vi "LSI336Data_initialize.vi"(0 "LSI336Data in":refnum<class "LSI336Data.lvclass">, 1 "RunName":string, 2 "InstName":string, 3 "FileFormat":string, 5 "LSI336Settings(X, Y)":T2(array[cluster])=[{"LSIName"="LSI218A", "Labels"=["N.C.", "N.C.", "N.C.", "N.C.", "N.C.", "N.C.", "N.C.", "N.C."], "SensorLocations"=[enum."N.C.", enum."N.C.", enum."N.C.", enum."N.C.", enum."N.C.", enum."N.C.", enum."N.C.", enum."N.C."], "Active?"=FALSE, "VISA res. name"=""}, {"LSIName"="LSI218B", "Labels"=["N.C.", "N.C.", "N.C.", "N.C.", "N.C.", "N.C.", "N.C.", "N.C."], "SensorLocations"=[enum."N.C.", enum."N.C.", enum."N.C.", enum."N.C.", enum."N.C.", enum."N.C.", enum."N.C.", enum."N.C."], "Active?"=FALSE, "VISA res. name"=""}, {"LSIName"="LSI218C", "Labels"=["N.C.", "N.C.", "N.C.", "N.C.", "N.C.", "N.C.", "N.C.", "N.C."], "SensorLocations"=[enum."N.C.", enum."N.C.", enum."N.C.", enum."N.C.", enum."N.C.", enum."N.C.", enum."N.C.", enum."N.C."], "Active?"=FALSE, "VISA res. name"=""}, {"LSIName"="LSI218D", "Labels"=["N.C.", "N.C.", "N.C.", "N.C.", "N.C.", "N.C.", "N.C.", "N.C."], "SensorLocations"=[enum."N.C.", enum."N.C.", enum."N.C.", enum."N.C.", enum."N.C.", enum."N.C.", enum."N.C.", enum."N.C."], "Active?"=FALSE, "VISA res. name"=""}, {"LSIName"="LSI218E", "Labels"=["N.C.", "N.C.", "N.C.", "N.C.", "N.C.", "N.C.", "N.C.", "N.C."], "SensorLocations"=[enum."N.C.", enum."N.C.", enum."N.C.", enum."N.C.", enum."N.C.", enum."N.C.", enum."N.C.", enum."N.C."], "Active?"=FALSE, "VISA res. name"=""}, {"LSIName"="LSI218F", "Labels"=["N.C.", "N.C.", "N.C.", "N.C.", "N.C.", "N.C.", "N.C.", "N.C."], "SensorLocations"=[enum."N.C.", enum."N.C.", enum."N.C.", enum."N.C.", enum."N.C.", enum."N.C.", enum."N.C.", enum."N.C."], "Active?"=FALSE, "VISA res. name"=""}], 9 "RUN start time":timestamp, 11 "error in (no error)":errorcluster, 12 "base path":path) -> (4 "LSI336Data out":refnum<class "LSI336Data.lvclass">, 6 "Status":T1(ring), 10 "AllLabels":string[](array[string]), 15 "error out":errorcluster)   [LabVIEW 2017, in "LSI336Data.lvclass"]
uses:
  LSI336Data.lvclass
  LSI336Data.lvclass/LSI336Data.ctl
  istr.lib/Lake Shore 336/Lake Shore 336.lvlib
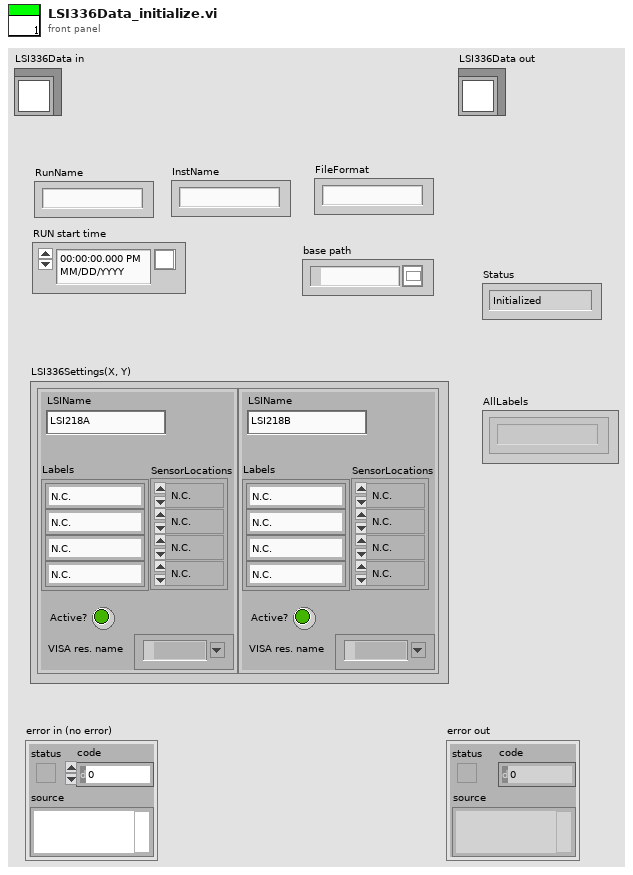
[diagram p1: front panel]
types:
  T1 = enum16{"Initialized", "Ready", "Measuring", "Terminated"}
  T2 = cluster{"LSIName":string, "Labels":string[], "SensorLocations":enum16{"N.C.", "T3He1-1", "T3He1-2", "T3He1-3", "T3He1-4", "T3He2-1", "T3He2-2", "T3He3", "T3He4", "T3He5", "T3He6-1", "T3He6-2", "T3He7-1", "T3He7-2", "T3He8", "T3He9", "T3He10", "T4He1", "T4He2-1", "T4He2-2", "T4He3-1", "T4He3-2", "T4He3-3", "T4He3-4", "T4He4", "T4He5", "T4He6", "T4He7", "T4He8", "T4He9", "T4He10", "T1K1", "T1K2", "T1K3-1", "T1K3-2", "T1K4", "T1K5", "T1K6", "TIP1", "TIP2", "TIP3", "TIP4", "TIP5", "TIP6", "TIP7", "TTH1", "TTH2", "TTH3", "TTH4"}[], "Active?":bool, "VISA res. name":refnum<visa-resource-name>}[]
  T3 = enum16{"open", "replace", "create", "open or create", "replace or create", "replace or create with confirmation"}
  T4 = cluster{"LSIName":string, "Labels":string[], "SensorLocations":enum16{"N.C.", "T3He1-1", "T3He1-2", "T3He1-3", "T3He1-4", "T3He2-1", "T3He2-2", "T3He3", "T3He4", "T3He5", "T3He6-1", "T3He6-2", "T3He7-1", "T3He7-2", "T3He8", "T3He9", "T3He10", "T4He1", "T4He2-1", "T4He2-2", "T4He3-1", "T4He3-2", "T4He3-3", "T4He3-4", "T4He4", "T4He5", "T4He6", "T4He7", "T4He8", "T4He9", "T4He10", "T1K1", "T1K2", "T1K3-1", "T1K3-2", "T1K4", "T1K5", "T1K6", "TIP1", "TIP2", "TIP3", "TIP4", "TIP5", "TIP6", "TIP7", "TTH1", "TTH2", "TTH3", "TTH4"}[], "Active?":bool, "VISA res. name":refnum<visa-resource-name>}
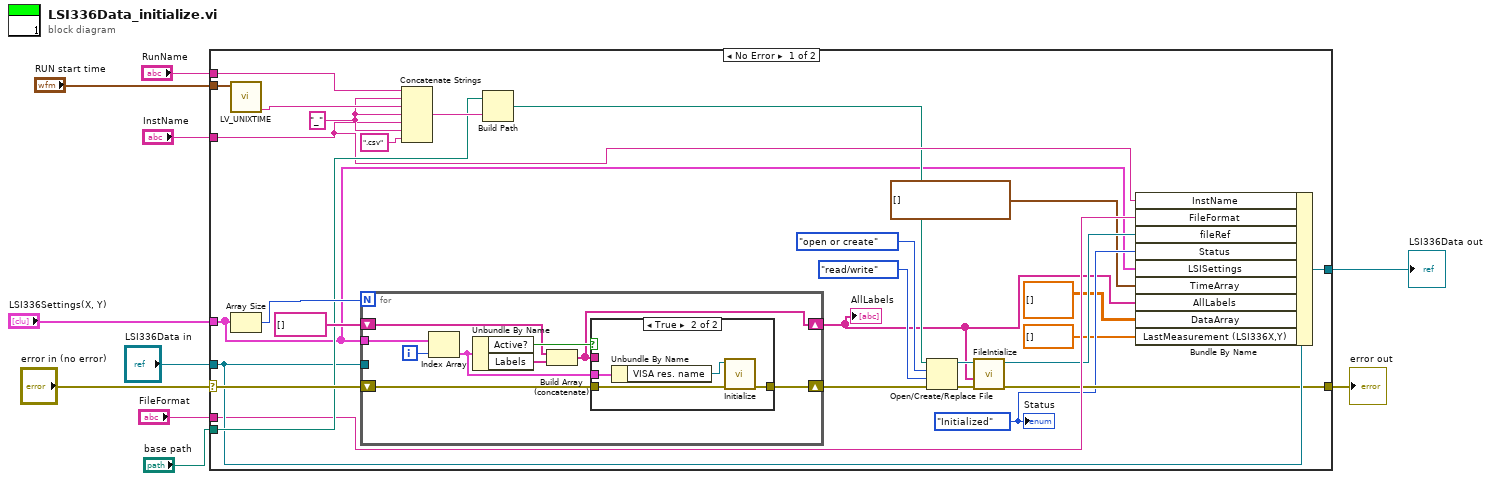
[diagram p0: block diagram]
diagram:
  n1 = case shown="No Error" "error in (no error)" {
    selector: "error in (no error)" -> [w38 w54]
    tunnel: [w20 w54] -> w9
    tunnel: [w17 w53] -> w7
    tunnel: "LSI336Data in" -> [w27 w53]
    tunnel: "LSI336Settings(X, Y)" -> [w15 _]
    tunnel: "RunName" -> [w34 _]
    tunnel: "RUN start time" -> [w33 _]
    tunnel: "InstName" -> [w26 _]
    tunnel: "base path" -> [w28 _]
    tunnel: "FileFormat" -> [w25 _]
    frame No Error {
      w16 = T1."Initialized" ("Status")
      w31 = "_" ("string")
      n2 = call "LV_UNIXTIME.vi"("current time"=w33) -> ("date/time string"=w32:string)  [unwired: 9 in, 1 out]
      n3 = Array Size(array=w15) -> (size(s)=w36:i32)
      n4 = for {
        N: w36 -> [_]
        shift-right: [w42] -> w14
        shift-left: string[] [] -> [w43]
        shift-right: [w39] -> w35
        shift-left: w38 -> [w40]
        tunnel: w27 -> [_]
        tunnel: w15 -> [w46]
        i -> [w47]
        n5 = Index Array(array=w46, index=w47) -> (element=w41:T4)
        n6 = Unbundle By Name(w41) -> ("Active?"=w45:bool, "Labels"=w44:string[])
        n7 = Build Array (concatenate)(w43, w44) -> (w42:string[])
        n8 = case shown="True" w45 {
          tunnel: w42 -> [_ _]
          tunnel: w41 -> [_ w51]
          tunnel: w40 -> [w48 w50]
          tunnel: [w48 w49] -> w39
          frame False {
          }
          frame True {
            n9 = Unbundle By Name(w51) -> ("VISA res. name"=w52:refnum<visa-resource-name>)
            n10 = call "Initialize.vi"("error in (no error)"=w50, "VISA resource name"=w52) -> ("error out"=w49:errorcluster)  [unwired: 8 in, 1 out]
          }
        }
      }
      "AllLabels" <- w14
      n11 = Concatenate Strings(w34, w31, w32, w31, w26, w31, ".csv" ("string")) -> (w29:string)
      n12 = Build Path(base path=w28, name or relative path=w29) -> (appended path=w24:path)
      n13 = Open/Create/Replace File(file path (use dialog)=w24, error in=w35, operation (0:open)=T3."open or create", access (0:read/write)=enum16{"read/write", "read-only", "write-only"}."read/write") -> (refnum out=w22:refnum<file>, error out=w19:errorcluster)  [unwired: 2 in, 1 out]
      n14 = call "FileIntialize.vi"("Error In"=w19, "Labels"=w14, "refnum in"=w22) -> ("Error Out"=w20:errorcluster, "File Refnum"=w21:refnum<file>)  [unwired: 7 in]
      n15 = Bundle By Name(cluster=w27, "InstName"=w26, "FileFormat"=w25, "fileRef"=w21, "Status"=w16, "LSISettings"=w15, "TimeArray"=timestamp[] [], "AllLabels"=w14, "DataArray"=dbl[][] [], "LastMeasurement (LSI336X,Y)"=dbl[] [] ("LastMeasurement (LSI336A-F)")) -> (w17:refnum<class "LSI336Data.lvclass">)
      "Status" <- w16
    }
    frame Error {
    }
  }
  "error out" <- w9
  "LSI336Data out" <- w7
